vi "Handle Last Ack Core.vi"(4 "error in (no error)":errorcluster, 6 "Last Ack":refnum<class "Last Ack.lvclass">, 7 "UI_Actor in":refnum<class "UI_Actor.lvclass">) -> (0 "error out":errorcluster, 3 "UI_Actor out":refnum<class "UI_Actor.lvclass">)   [LabVIEW 2020, in "UI_Actor.lvlib" / "UI_Actor.lvclass"]
doc: "(<B>Filename</B>: Actor Framework.lvlib:Actor.lvclass:Handle Last Ack Core.vi)\n\nDefines how the caller actor responds to the Last Ack message from a nested actor. The Last Ack message is the final message a nested actor sends to its caller before it shuts down. The message contains information about the final state of the nested actor.\n\nBy default, this method does nothing except return any error the nested actor sent. A descendant class may override this method to define behavior."
uses:
  UI_Actor.lvclass
  support/Actor Framework.lvlibp/1abvi3w/vi.lib/ActorFramework/LastAck/Last Ack.lvclass
  D:/Projets/STEP AT/UI Actor/support/Actor Framework.lvlibp/1abvi3w/vi.lib/ActorFramework/Actor/Actor.lvclass
  UI_Actor.lvclass/UI_Actor.ctl
  support/Actor Framework.lvlibp/1abvi3w/vi.lib/ActorFramework/Actor/Actor.lvclass
  support/Actor Framework.lvlibp/1abvi3w/vi.lib/ActorFramework/Stop Msg/Stop Msg.lvclass
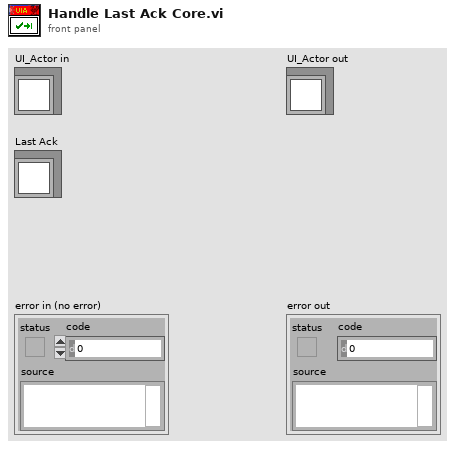
[diagram p1: front panel]
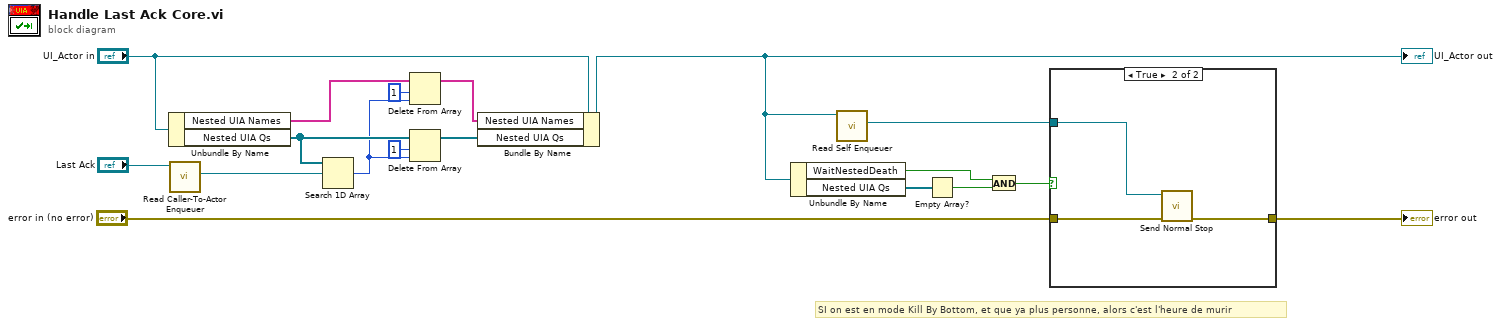
[diagram p0: block diagram]
diagram:
  # "SI on est en mode Kill By Bottom, et que ya plus personne, alors c'est l'heure de murir"
  n1 = Unbundle By Name("UI_Actor in") -> ("Nested UIA Names"=w11:string[], "Nested UIA Qs"=w13:refnum<class "Message Enqueuer.lvclass">[])
  n2 = call "Read Caller-To-Actor Enqueuer.vi"("Last Ack"="Last Ack") -> ("Caller-to-Actor Enqueuer"=w16:refnum<class "Message Enqueuer.lvclass">)  [unwired: 10 in]
  n3 = Search 1D Array(1D array=w13, element=w16) -> (index of element=w9:i32)  [unwired: 1 in]
  n4 = Delete From Array(array=w11, length=1, index=w9) -> (array with subset deleted=w10:string[])  [unwired: 1 out]
  n5 = Delete From Array(array=w13, length=1, index=w9) -> (array with subset deleted=w15:refnum<class "Message Enqueuer.lvclass">[])  [unwired: 1 out]
  n6 = Bundle By Name(cluster="UI_Actor in", "Nested UIA Names"=w10, "Nested UIA Qs"=w15) -> (w5:refnum<class "UI_Actor.lvclass">)
  "UI_Actor out" <- w5
  n7 = Unbundle By Name(w5) -> ("WaitNestedDeath"=w3:bool, "Nested UIA Qs"=w4:refnum<class "Message Enqueuer.lvclass">[])
  n8 = call "Read Self Enqueuer.vi"("Actor"=w5) -> ("Self Enqueuer"=w8:refnum<class "Message Enqueuer.lvclass">)  [unwired: 10 in]
  n9 = Empty Array?(array=w4) -> (empty?=w2:bool)
  n10 = And(x=w3, y=w2) -> (x .and. y?=w1:bool)
  n11 = case shown="True" w1 {
    tunnel: w8 -> [_ w22]
    tunnel: "error in (no error)" -> [w19 w21]
    tunnel: [w19 w20] -> w6
    frame False {
    }
    frame True {
      n12 = call "Send Normal Stop.vi"("error in (no error)"=w21, "Message Enqueuer"=w22) -> ("error out"=w20:errorcluster)  [unwired: 9 in]
    }
  }
  "error out" <- w6
